vi "XIPIN_IBERT_Spartan6_GTP_(ChipScope_Pro_-_IBERT)_2_02_a.vi"   [LabVIEW 2017]
doc: "The ChipScope(TM) Pro Integrated Bit Error Ratio Tester (IBERT) core for Spartan(R)-6 GTP is a customizable core that can be used to evaluate and monitor the health of Spartan-6 GTP Transceivers.\n------------------------------------\n<b>Need License</b> : No"
uses:
  <vilib>/rvi/XilinxIP/XIPIN_XNode/niFpgaXIPIN.xnode
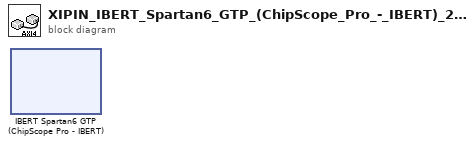
[diagram p0: block diagram]
diagram:
  n1 = xnode ("IBERT Spartan6 GTP (ChipScope Pro - IBERT)")() -> ()
